vi "RespHeaderToString.vi"(11 "Headers":T1) -> (3 "HeaderString":string)   [LabVIEW 2020, in "net-http-client.lvclass"]
uses:
  net-http-client.lvclass
  net-http-client.lvclass/net-http-client.ctl
  <vilib>/Viviota/Viviota HTTP Client NET/HTTPHeaders_NET/HttpHeaders_NET.lvclass
  <vilib>/Viviota/Viviota HTTP Client NET/HttpHeaders_response/HttpHeaders_Response.lvclass
  C:/Program Files/National Instruments/LabVIEW 2020/vi.lib/Viviota/Viviota HTTP Client NET/HTTPHeaders_NET/HttpHeaders_NET.lvclass
  C:/Program Files/National Instruments/LabVIEW 2020/vi.lib/Viviota/Viviota HTTP Client NET/HttpHeaders_response/HttpHeaders_Response.lvclass
  <vilib>/Viviota/Viviota HTTP Client NET/HttpHeaders_content/HttpHeaders_Content.lvclass
  C:/Program Files/National Instruments/LabVIEW 2020/vi.lib/Viviota/Viviota HTTP Client NET/HttpHeaders_content/HttpHeaders_Content.lvclass
  <vilib>/Viviota/Viviota HTTP Client NET/Types/ResponseHeaders_Cluster.ctl
  <vilib>/Viviota/Viviota HTTP Client NET/HttpClient_NET.lvlib
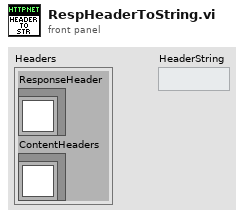
[diagram p1: front panel]
types:
  T1 = typedef "HttpClient_NET.lvlib/ResponseHeaders_Cluster.ctl" = cluster{"ResponseHeader":refnum<class "HttpHeaders_Response.lvclass">, "ContentHeaders":refnum<class "HttpHeaders_Content.lvclass">}
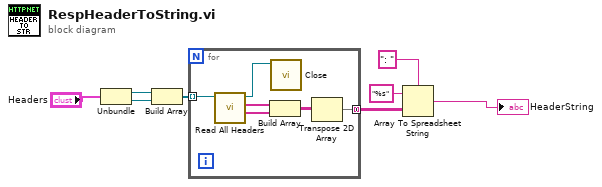
[diagram p0: block diagram]
diagram:
  n1 = Unbundle("Headers") -> ("ResponseHeader"=w3:refnum<class "HttpHeaders_Response.lvclass">, "ContentHeaders"=w2:refnum<class "HttpHeaders_Content.lvclass">)
  n2 = Build Array(w3, w2) -> (w4:refnum<class "HttpHeaders_NET.lvclass">[])
  n3 = for {
    tunnel: w4 -> [w14] mode=indexing
    tunnel: [w10] -> w5 mode=concatenating
    n4 = call-dynamic "Read All Headers.vi"("HTTPHeaders_NET in"=w14) -> ("Header Values"=w12:string[], "Header Names"=w13:string[], "HTTPHeaders_NET out"=w9:refnum<class "HttpHeaders_NET.lvclass">)  [unwired: 7 in, 1 out]
    n5 = Build Array(w13, w12) -> (w11:string[][])
    n6 = call <vilib>:"Close.vi"("HTTPHeaders_NET in"=w9) -> ()  [unwired: 10 in, 1 out]
    n7 = Transpose 2D Array(2D array=w11) -> (transposed array=w10:string[][])
  }
  n8 = Array To Spreadsheet String(delimiter (Tab)=": ", array=w5, 3:"%s" ("format string")) -> (spreadsheet string=→"HeaderString":string)
